vi "testParseStateQueueEmptyString.vi"(8 "error in (no error)":errorcluster, 11 "testStateMachineUtilities in":refnum<class "testStateMachineUtilities.lvclass">) -> (0 "error out":errorcluster, 3 "testStateMachineUtilities out":refnum<class "testStateMachineUtilities.lvclass">)   [LabVIEW 2013, in "testStateMachineUtilities.lvclass"]
uses:
  testStateMachineUtilities.lvclass
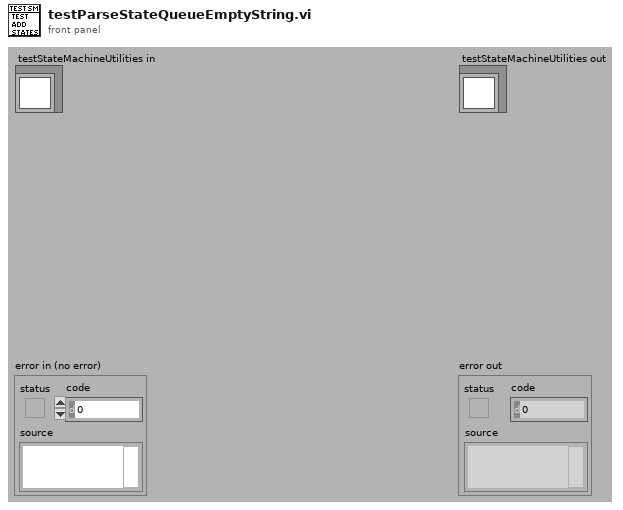
[diagram p1: front panel]
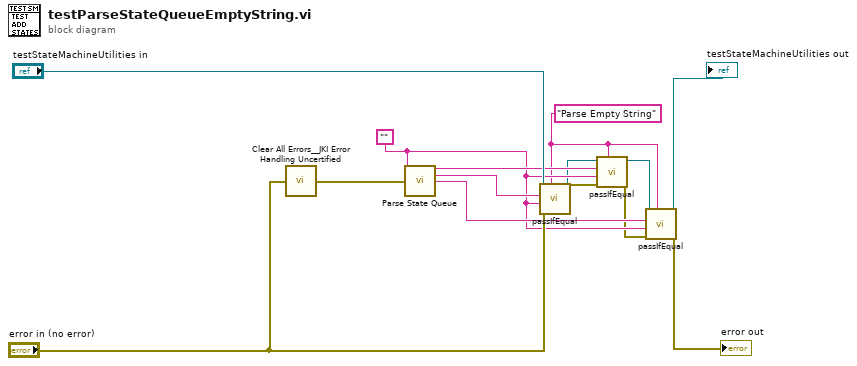
[diagram p0: block diagram]
diagram:
  w1 = "Parse Empty String" ("custom report message (\"\")")
  w7 = "" ("State Queue")
  n1 = call <vilib>:"Clear All Errors__JKI Error Handling Uncertified.vi"("error in"="error in (no error)") -> ("no error out"=w12:errorcluster)  [unwired: 4 in]
  n2 = call "Parse State Queue.vi"("State Queue"=w7, "Error In (no error)"=w12) -> ("Remaining States"=w10:string, "Current State"=w11:string, "Arguments"=w9:string)  [unwired: 11 in]
  n3 = call-dynamic "passIfEqual.vi"("custom report message (\"\")"=w1, "error in (no error)"="error in (no error)", "y"=w7, "x"=w11, "TestCase in"="testStateMachineUtilities in") -> ("error out"=w4:errorcluster, "TestCase out"=w5:refnum<class "testStateMachineUtilities.lvclass">)  [unwired: 5 in]
  n4 = call-dynamic "passIfEqual.vi"("custom report message (\"\")"=w1, "error in (no error)"=w4, "y"=w7, "x"=w10, "TestCase in"=w5) -> ("error out"=w3:errorcluster, "TestCase out"=w8:refnum<class "testStateMachineUtilities.lvclass">)  [unwired: 5 in]
  n5 = call-dynamic "passIfEqual.vi"("custom report message (\"\")"=w1, "error in (no error)"=w3, "y"=w7, "x"=w9, "TestCase in"=w8) -> ("error out"=→"error out":errorcluster, "TestCase out"=→"testStateMachineUtilities out":refnum<class "testStateMachineUtilities.lvclass">)  [unwired: 5 in]
